vi "Unibot - State Machine Controller v2.vi"(4 "Parameters":T1={"Limit"=10.0, "Control Dead Band"=20.0, "Error Dead Band"=20.0}, 5 "Up Optimal Gain":dbl[](array[numeric])=[-16.4615, -16.2422, -3.1287, -2.0658], 6 "Mode":T2(ring), 7 "Setpoint":dbl(knob) scale=-1.0..1.0, 8 "Enable":bool, 9 "Kill":bool, 10 "PID gains":T3={"proportional gain (Kc)"=1.0, "integral time (Ti, min)"=0.01, "derivative time (Td, min)"=0.0} {"derivative time (Td, min)" format="%.3f"; "integral time (Ti, min)" format="%.3f"; "proportional gain (Kc)" format="%.3f"}, 11 "States":dbl[](array[numeric])=[-0.0012566370614359172, -0.8117875416876026, 0.0, 0.0]) -> (0 "Status":string="Kill", 2 "Control Effort":dbl(knob) scale=-1000.0..1000.0)   [LabVIEW 2012]
uses:
  Unibot - States.ctl
  <vilib>/Simulation/Scripting/Companion Diagram/SimConfigNode/SimParams.ctl
  <vilib>/Simulation/Scripting/Companion Diagram/SimConfigNode/_simSolvers.ctl
  <vilib>/Simulation/Implementation/Shared/SIMSCR Execution Mode.ctl
  <vilib>/Simulation/Param Hierarchy/Typedefs/SIMPH Param Control Actions.ctl
  <vilib>/Simulation/Implementation/Shared/NILVSim_ParamChanged.vi
  <vilib>/Simulation/Implementation/Shared/NILVSim_Manager.vi
  <vilib>/Simulation/Implementation/Shared/NILVSim_FinalizeModel.vi
  <vilib>/addons/Control Design/_Implementation/CD State Feedback Controller (Single Output).vi
  <vilib>/Simulation/Implementation/Shared/SIM Unbundle Sim Info.vi
  <vilib>/Utility/error.llb/Clear Errors.vi
  <vilib>/Simulation/Implementation/Shared/NILVSim_GetModelError.vi
  <vilib>/Simulation/Implementation/Shared/SIM Bundle Sim Info.vi
  <vilib>/Simulation/Implementation/Shared/NILVSim_Initialize.vi
  <vilib>/Simulation/Utility/Implementation/NILVSim Get Time and IsAcceptedStep.vi
  <vilib>/Simulation/Implementation/Shared/SIMSH Read Queue.vi
  <vilib>/Simulation/Implementation/XNodeFramework/SimXNode/SimX.xnode
  <vilib>/Simulation/Model Libraries/PID/SIM Advanced PID (Academic).vi
  <vilib>/Simulation/Scripting/Companion Diagram/SimConfigNode/SimDog.xnode
  <vilib>/addons/Control Design/_Implementation/NI_CD_Implementation.lvlib
  <vilib>/Simulation/Implementation/Shared/NI_SIM_Implementation.lvlib
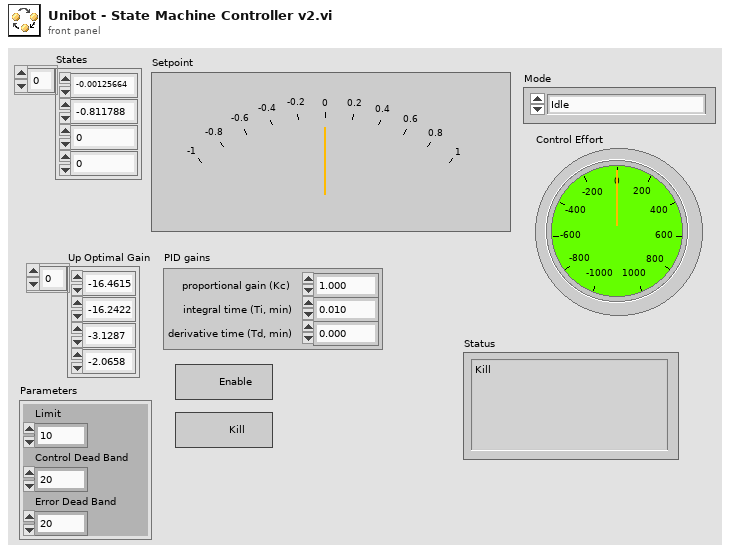
[diagram p1: front panel]
types:
  T1 = cluster{"Limit":dbl, "Control Dead Band":dbl, "Error Dead Band":dbl}
  T2 = enum16{"Idle", "Linear Balance", "Proportional Balance", "PID Balance", "Emergency"}
  T3 = cluster{"proportional gain (Kc)":dbl, "integral time (Ti, min)":dbl, "derivative time (Td, min)":dbl}
  T4 = typedef "Unibot - States.ctl" = enum16{"Idle", "Linear Balance", "Proportional Balance", "PID Balance", "Emergency"}
  T5 = enum16{"Simulate to Completion", "Single Time-Step Simulation (Fixed Step Only)"}
  T6 = typedef "SIMSCR Execution Mode.ctl" = enum16{"Simulate to Completion", "Single Time-Step Simulation (Fixed Step Only)"}
  T7 = typedef "SIMPH Param Control Actions.ctl" = enum16{"get params", "set params"}
  T8 = cluster{"SIMSH Sim Time":dbl, "Saturation 2":cluster{"output":dbl}, "Unbundle By Name":cluster{"output high":dbl, "output low":dbl}, "output range":cluster{"output high":dbl, "output low":dbl}, "Select 3":cluster{"s? t:f":dbl}, "Equal To 0?":cluster{"x = 0?":bool}, "Reciprocal":cluster{"1/x":dbl}, "Select 2":cluster{"s? t:f":dbl}, "Select":cluster{"s? t:f":dbl}, "Summation 3":cluster{"Result":dbl}, "Gain 2":cluster{"output":dbl}, "Summation 2":cluster{"Result":dbl}, "Subtract 3":cluster{"x-y":dbl}, "Subtract 2":cluster{"x-y":dbl}, "Multiply 2":cluster{"x*y":dbl}, "Subtract":cluster{"x-y":dbl}, "Multiply":cluster{"x*y":dbl}, "SIM PID Derivative Gain.vi":cluster{"output":dbl}, "SIM PID Derivative Gain.vi - SIMSH":cluster{"SIMSH Sim Time":dbl, "t 3":dbl, "Select 2":cluster{"s? t:f":dbl}, "Equal?":cluster{"x = y?":bool}, "Or":cluster{"x .or. y?":bool}, "Equal To 0?":cluster{"x = 0?":bool}}, "Gain":cluster{"output":dbl}, "Summation":cluster{"Result":dbl}, "Integral Gain - series.vi":cluster{"output":dbl}, "Integral Gain - series.vi - SIMSH":cluster{"SIMSH Sim Time":dbl, "Select 2":cluster{"s? t:f":dbl}, "integral in gain?":bool, "Integrator":cluster{"output y(k)":dbl}, "Gain 2":cluster{"output":dbl}, "Select":cluster{"s? t:f":dbl}, "Equal To 0?":cluster{"x = 0?":bool}, "Reciprocal":cluster{"1/x":dbl}}}
  T9 = typedef "SimParams.ctl" = cluster{"Initial Time (s)":dbl, "Final Time (s)":dbl, "Step Size (s)":dbl, "ODE Solver":T10, "Minimum Step Size (s)":dbl, "Maximum Step Size (s)":dbl, "Relative Tolerance":dbl, "Absolute Tolerance":dbl, "Software Timing":bool, "Initial Step Size (s)":dbl, "Automatic Fixed Step Size?":bool, "Automatic Discrete Step Size?":bool, "Discrete Step Size (s)":dbl, "Calculate using Time Step":bool, "Solver Wired?":bool, "Prev.Frm.Expected End":u64, "Prev.Frm.Actual End":u64, "Prev.Frm.Finished Late?":bool, "Prev.Iter.Expected End":u64, "Prev.Iter.Actual End":u64, "Prev.Iter.Finished Late?":bool, "Expected Iteration Start":u64, "Actual Iteration Start":u64, "Expected Frame Start":u64, "Actual Frame Start":u64, "Source Name":string, "Name":string, "Period":i64, "Deadline":i64, "Offset":i64, "Start":i64, "Priority":i32, "Timeout":i32, "Processor":i32, "Mode":enum32{"No Change", "Process missed periods, maintain original phase", "Discard missed periods, maintain original phase", "Process missed periods, ignore original phase", "Discard missed periods, ignore original phase"}, "Wakeup reason":enum32{"Normal", "Aborted", "Asynchronous wakeup", "Timing source error", "Timed loop error", "Timeout"}, "Error":errorcluster, "Source Type":string, "Secondary Source Type":string, "Global End Time":u64, "Global Start Time":u64, "Full Solver Reset":bool, "Execution Mode":T6, "Nan/Inf Check":bool, "Custom Solver Library":string, "Solver Is Variable":bool, "custom solver name":string, "Signal Collection Decimation":u32}
  T10 = typedef "_simSolvers.ctl" = enum16{"Runge-Kutta 1 (Euler)", "Runge-Kutta 2", "Runge-Kutta 3", "Runge-Kutta 4", "Runge-Kutta 23 (variable)", "Runge-Kutta 45 (variable)", "BDF (variable)", "Adams-Moulton (variable)", "Rosenbrock (variable)", "Discrete States Only", "SDIRK 4 (variable)", "Radau 5 (variable)", "Radau 9 (variable)", "Radau 13 (variable)", "Radau [Variable Order] (variable)", "Gear's Method (variable)", "Linearizer", "State Query", "Trim Eval", "Custom Solver"}
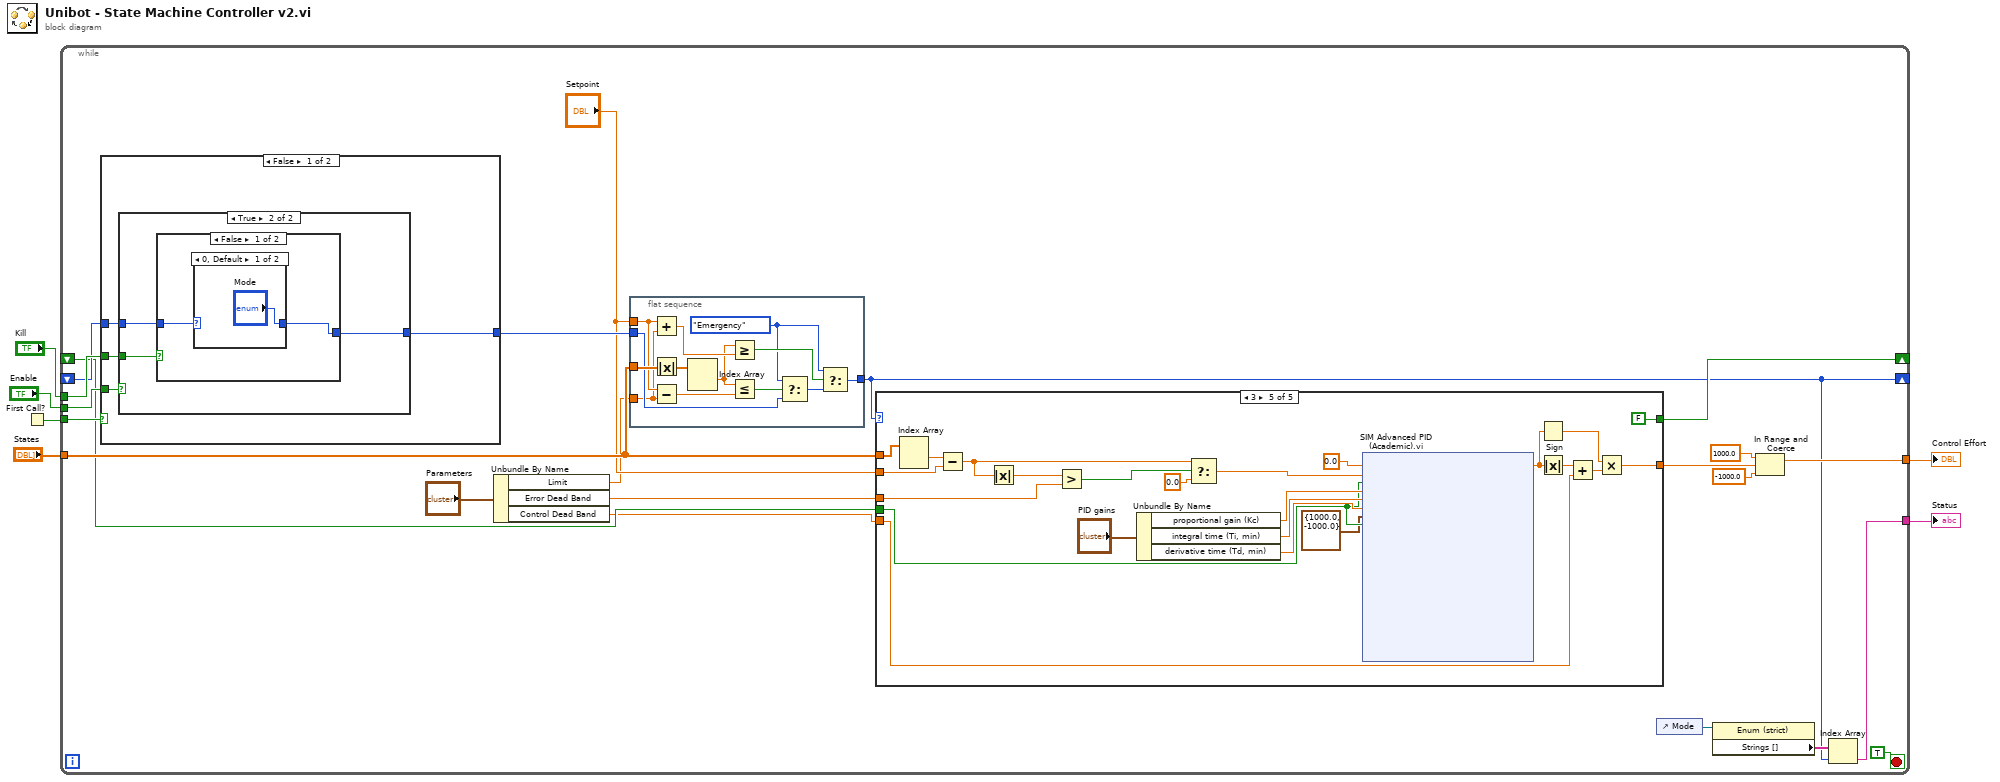
[diagram p0: block diagram]
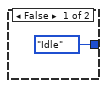
[diagram p2: hidden frame]
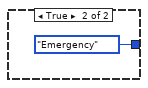
[diagram p4: hidden frame]
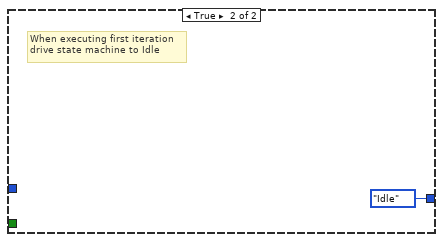
[diagram p5: hidden frame]
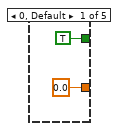
[diagram p6: hidden frame]
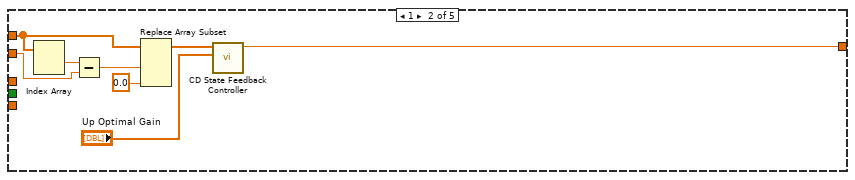
[diagram p7: hidden frame]
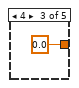
[diagram p8: hidden frame]
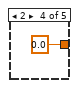
[diagram p9: hidden frame]
diagram:
  n1 = First Call?() -> (First Call?: T/F=w3:bool)
  n2 = while {
    tunnel: "States" -> [w23]
    tunnel: [w20] -> w1
    shift-right: [w12] -> _
    shift-left: _ -> [w26]
    tunnel: [w16] -> w5
    tunnel: "Kill" -> [w27]
    tunnel: w3 -> [w25]
    tunnel: "Enable" -> [w24]
    shift-right: [w14] -> _
    shift-left: _ -> [w15]
    stop <- TRUE stop-if-true
    n3 = case shown="False" w25 {
      tunnel: w27 -> [w45 _]
      tunnel: w26 -> [w44 _]
      tunnel: w24 -> [w43 _]
      tunnel: [w42 Unibot_-_States."Idle" ("Enum")] -> w22
      frame False {
        n4 = case shown="True" w43 {
          tunnel: w45 -> [_ w49]
          tunnel: w44 -> [_ w47]
          tunnel: [Unibot_-_States."Idle" ("Enum") w48] -> w42
          frame False {
          }
          frame True {
            n5 = case shown="False" w49 {
              tunnel: [w50 Unibot_-_States."Emergency" ("Enum")] -> w48
              tunnel: w47 -> [w51 _]
              frame False {
                n6 = case shown="0, Default" w51 {
                  selector: w51 -> [_ w53]
                  tunnel: ["Mode" w53] -> w50
                  frame 0, Default {
                  }
                  frame 4 {
                  }
                }
              }
              frame True {
              }
            }
          }
        }
      }
      frame True {
        # "When executing first iteration\ndrive state machine to Idle"
      }
    }
    n7 = Unbundle By Name("Parameters") -> ("Limit"=w9:dbl, "Error Dead Band"=w8:dbl, "Control Dead Band"=w7:dbl)
    n8 = flat-sequence {
      tunnel: w23 -> [w39]
      tunnel: w22 -> [w32]
      tunnel: [w41] -> w12
      tunnel: "Setpoint" -> [w37]
      tunnel: w9 -> [w29]
      frame #0 {
        w31 = Unibot_-_States."Emergency" ("Enum")
        n9 = Add(x=w37, y=w29) -> (x+y=w35:dbl)
        n10 = Absolute Value(x=w39) -> (abs(x)=w40:dbl[])
        n11 = Subtract(x=w37, y=w29) -> (x-y=w36:dbl)
        n12 = Index Array(array=w40) -> (element #1=w30:dbl)  [unwired: 2 in, 1 out]
        n13 = Greater Or Equal?(x=w30, y=w35) -> (x >= y?=w34:bool)
        n14 = Less Or Equal?(x=w30, y=w36) -> (x <= y?=w38:bool)
        n15 = Select(t=w31, s=w38, f=w32) -> (s? t:f=w33:i32)
        n16 = Select(t=w31, s=w34, f=w33) -> (s? t:f=w41:i32)
      }
    }
    n17 = case shown="3" w12 {
      tunnel: w23 -> [_ w62 _ _ w90]
      tunnel: [0.0 w60 0.0 0.0 ("output") w87] -> w21
      tunnel: "Setpoint" -> [_ w59 _ _ w77]
      tunnel: w15 -> [_ _ _ _ w71]
      tunnel: [TRUE ("Enable") _ _ _ FALSE ("Enable")] -> w14
      tunnel: w7 -> [_ _ _ _ w88]
      tunnel: w8 -> [_ _ _ _ w80]
      frame 0, Default {
      }
      frame 1 {
        n18 = Index Array(array=w62) -> (element #1=w61:dbl)  [unwired: 2 in, 1 out]
        n19 = Subtract(x=w61, y=w59) -> (x-y=w64:dbl)
        n20 = Replace Array Subset(array=w62, new element #1=w64, new element #2=0.0 ("x")) -> (w65:dbl[])  [unwired: 2 in]
        n21 = call-poly <vilib>:"CD State Feedback Controller.vi"("Controller Gain"="Up Optimal Gain", "States"=w65) -> ("Controller Action"=w60:dbl)  [unwired: 1 in, 8 out]
      }
      frame 4 {
      }
      frame 2 {
      }
      frame 3 {
        n22 = Index Array(array=w90) -> (element #1=w78:dbl)  [unwired: 2 in, 1 out]
        n23 = Subtract(x=w78, y=w77) -> (x-y=w79:dbl)
        n24 = Absolute Value(x=w79) -> (abs(x)=w81:dbl)
        n25 = Greater?(x=w81, y=w80) -> (0:w82:bool)
        n26 = Unbundle By Name("PID gains") -> ("proportional gain (Kc)"=w74:dbl, "integral time (Ti, min)"=w73:dbl, "derivative time (Td, min)"=w72:dbl)
        n27 = Select(t=w79, s=w82, f=0.0) -> (s? t:f=w76:dbl)
        n28 = xnode "SIM Advanced PID (Academic).vi"("Setpoint"=0.0, "Measurement"=w76, "Initialize?"=w71, "Proportional Gain (Kc)"=w74, "Integral time [s] (Ti)"=w73, "Derivative time [s] (Td)"=w72, "output range"=cluster{"output high":dbl, "output low":dbl} {"output high"=1000.0, "output low"=-1000.0}, "Initialize"=w71) -> ("Output"=w70:dbl)  [unwired: 1 in, 1 out]
        n29 = Sign(1:w70) -> (0:w85:dbl)
        n30 = Absolute Value(x=w70) -> (abs(x)=w86:dbl)
        n31 = Add(x=w86, y=w88) -> (x+y=w84:dbl)
        n32 = Multiply(x=w85, y=w84) -> (x*y=w87:dbl)
      }
    }
    n33 = control-ref of="Mode"() -> (w13:refnum<vi>)
    n34 = property class="Enum (strict)"(reference=w13) -> ("Strings []"=w17:string[])  [unwired: 1 in, 2 out]
    n35 = In Range and Coerce(upper limit=1000.0, x=w21, lower limit=-1000.0) -> (coerced(x)=w20:dbl)  [unwired: 1 out]
    n36 = Index Array(array=w17, index=w12) -> (element=w16:string)
  }
  "Control Effort" <- w1
  "Status" <- w5
